vi "escala.vi"() -> ()   [LabVIEW 2017]
panel:
  out "Tempo (s)":dbl
  out "Temperatura":dbl(slide) scale=0.0..212.0
  in  "Escala":bool
  # "ºF"
  # "ºC"
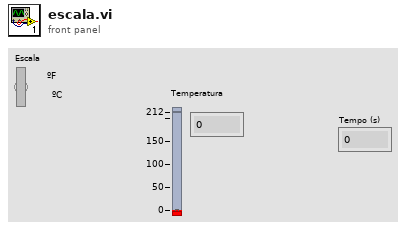
[diagram p1: front panel]
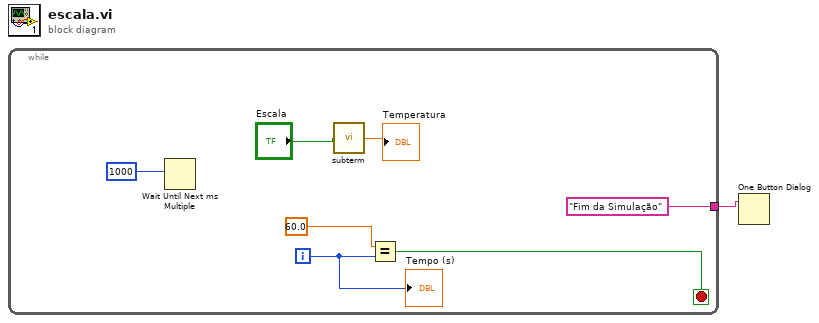
[diagram p0: block diagram]
diagram:
  n1 = while {
    tunnel: ["Fim da Simulação"] -> w1
    i -> [w4]
    stop <- w6 stop-if-true
    n2 = Wait Until Next ms Multiple(millisecond multiple=1000) -> ()  [unwired: 1 out]
    n3 = call "subterm.vi"("Escala"="Escala") -> ("Temperatura"=→"Temperatura":dbl)
    n4 = Equal?(x=60.0, y=w4) -> (x = y?=w6:bool)
    "Tempo (s)" <- w4
  }
  n5 = One Button Dialog(message=w1) -> ()  [unwired: 1 in, 1 out]
